vi "XTicks2003.vi"   [LabVIEW 2013]
uses:
  ModeType.ctl
  <vilib>/Heliosphere Research LLC/Advanced Plotting Toolkit/Advanced Plotting Toolkit.lvlib
types:
  T1 = typedef "ModeType.ctl" = enum16{"Normal", "Expected Failure", "Skipped", "Broken"}
  T2 = typedef "Advanced Plotting Toolkit.lvlib/PlotID.ctl" = i32
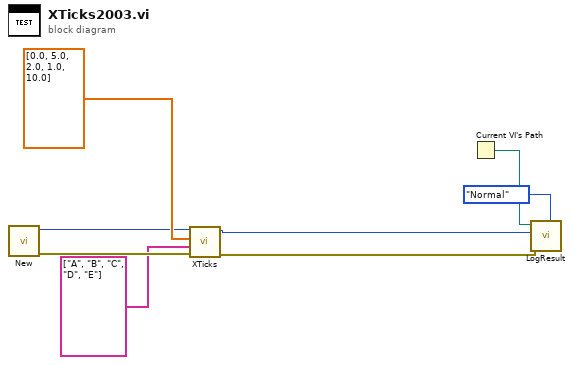
[diagram p0: block diagram]
diagram:
  n1 = call <vilib>:"New.vi"() -> ("error out"=w5:errorcluster, "Plot ID"=w6:T2)  [unwired: 10 in]
  n2 = call <vilib>:"XTicks.vi"("error in (no error)"=w5, "Tick Labels"=string[] ["A", "B", "C", "D", "E"], "Tick Locations"=dbl[] [0.0, 5.0, 2.0, 1.0, 10.0], "Plot ID"=w6) -> ("error out"=w4:errorcluster, "Plot ID Out"=w3:T2)  [unwired: 6 in]
  n3 = Current VI's Path() -> (path=w8:path)
  n4 = call "LogResult.vi"("Mode"=ModeType."Normal", "Test Result"=w4, "Test Artifact"=w3, "VI Path"=w8) -> ()  [unwired: 8 in]
